vi "Condition Step Configuration.vi"(8 "error in (no error)":errorcluster, 10 "Parameters In":variant, 11 "Subpanel Queue In":refnum<queue>) -> (0 "error out":errorcluster, 2 "Parameters Out":variant)   [LabVIEW 2018]
doc: "Configuration control for the 'Wait for Condition' step."
uses:
  controls/Condition Cluster.ctl
panel:
  in  "Condition parameters":T1
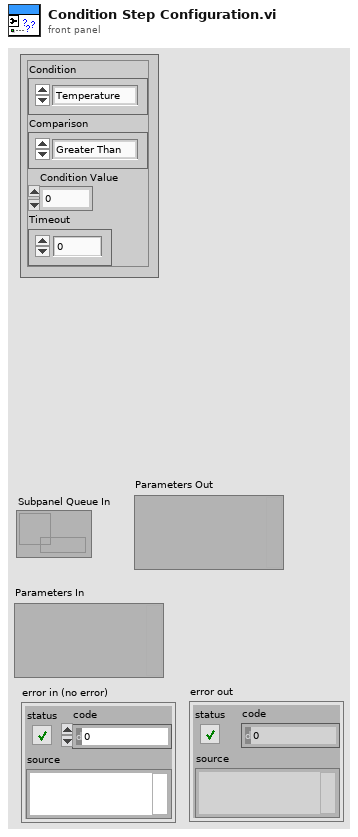
[diagram p1: front panel]
types:
  T1 = typedef "Condition Cluster.ctl" = cluster{"Condition":enum16{"Temperature", "pH", "Digital Trigger"}, "Comparison":enum16{"Greater Than", "Less Than", "Equal"}, "Condition Value":dbl, "Timeout":dbl}
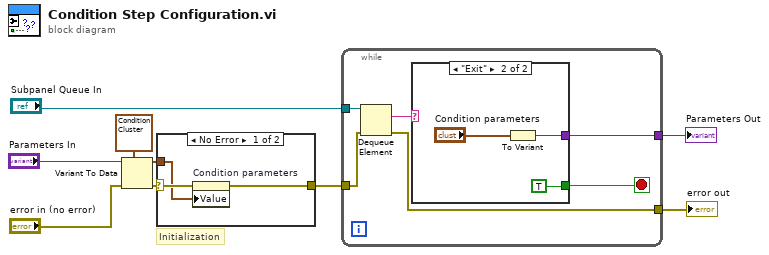
[diagram p0: block diagram]
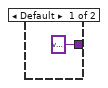
[diagram p2: hidden frame]
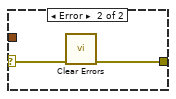
[diagram p3: hidden frame]
diagram:
  # "Initialization"
  n1 = Variant To Data(error in="error in (no error)", type=T1 {"Condition"=enum."Temperature", "Comparison"=enum."Greater Than", "Condition Value"=0.0, "Timeout"=0.0} ("Condition parameters"), Variant="Parameters In") -> (data=w8:T1, error out=w7:errorcluster)
  n2 = case shown="No Error" w7 {
    selector: w7 -> [w12 w14]
    tunnel: w8 -> [w11 _]
    tunnel: [w10 w13] -> w5
    frame No Error {
      n3 = property on="Condition parameters" class="Clust (strict)"(error in=w12, "Value"=w11) -> (error out=w10:errorcluster)  [unwired: 1 in, 1 out]
    }
    frame Error {
      n4 = call <vilib>:"Clear Errors.vi"("error in (no error)"=w14) -> ("error out"=w13:errorcluster)  [unwired: 5 in, 1 out]
    }
  }
  n5 = while {
    tunnel: "Subpanel Queue In" -> [w19]
    tunnel: w5 -> [w18]
    tunnel: [w17] -> w3
    tunnel: [w15] -> w1
    stop <- w16 stop-if-true
    n6 = Dequeue Element(queue=w19, error in (no error)=w18) -> (element=w20:string, error out=w15:errorcluster)  [unwired: 1 in, 2 out]
    n7 = case shown="\"Exit\"" w20 {
      tunnel: [variant ("Variant") w24] -> w17
      tunnel: [_ TRUE] -> w16
      frame Default {
      }
      frame "Exit" {
        n8 = To Variant(anything="Condition parameters") -> (Variant=w24:variant)
      }
    }
  }
  "Parameters Out" <- w3
  "error out" <- w1
